vi "Low Pass Filter.vi"(0 "input signal":waveform(dbl)={"t0"=timestamp(0 s since 1904-01-01), "dt"=0.0, "Y"=[]}, 1 "Lower Cutoff Frequency (Hz)":dbl=1000.0 format="%#_15g", 3 "Upper Cutoff Frequency (Hz)":dbl=200.0 format="%#_15g", 5 "error in":errorcluster, 7 "reset":bool) -> (14 "filtered data":waveform(dbl), 19 "error out":errorcluster)   [LabVIEW 2014]
doc: "Filters a time signal using an infinite impulse response (IIR) or finite impulse response (FIR) filter. Use this step to remove or attenuate unwanted frequencies from a signal using various standard filter types and topologies.\n\nThis Express VI filters the input signal continuously. The Express VI resets the signal to its original value the first time the Express VI runs, if LabVIEW detects a discontinuity in the input signal, or if the <b>reset</b> input receives a TRUE value."
uses:
  <vilib>/measure/macond.llb/IIR Filter for 1 Chan.vi
  <vilib>/measure/NI_MAPro.lvlib
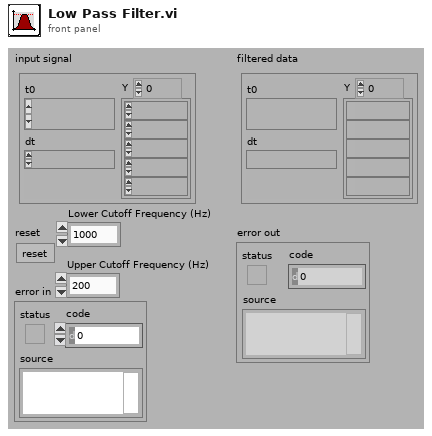
[diagram p1: front panel]
types:
  T1 = cluster{"Topology":enum16{"Off", "Butterworth", "Chebyshev", "Inverse Chebyshev", "Elliptic", "Bessel"}, "Type":enum16{"Lowpass", "Highpass", "Bandpass", "Bandstop"}, "Order":i32, "Lower Fc":dbl, "Upper Fc":dbl, "PB Ripple":dbl, "SB Attenuation":dbl}
  T2 = cluster{"Lower PB":dbl, "Upper PB":dbl, "Lower SB":dbl, "Upper SB":dbl, "PB Gain":dbl, "SB Gain":dbl, "Scale":bool}
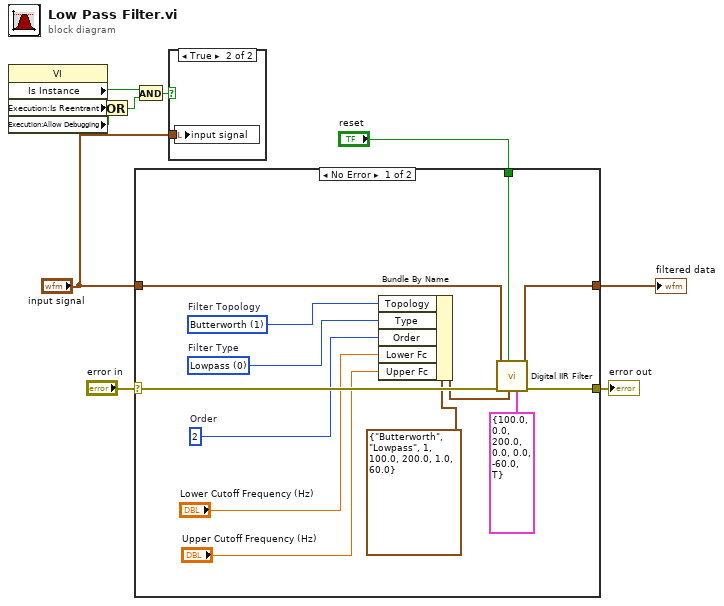
[diagram p0: block diagram]
diagram:
  n1 = property class="VI"() -> ("Is Instance"=w6:bool, "Execution:Is Reentrant"=w4:bool, "Execution:Allow Debugging"=w3:bool)  [unwired: 2 in, 2 out]
  n2 = Or(x=w4, y=w3) -> (x .or. y?=w5:bool)
  n3 = case shown="No Error" "error in" {
    selector: "error in" -> [w20 w24]
    tunnel: [w23 w24] -> w10
    tunnel: [w22 _] -> w8
    tunnel: "input signal" -> [w21 _]
    tunnel: "reset" -> [w19 _]
    frame No Error {
      w16 = u32 2  # Order
      w17 = u16 0 items=["Lowpass", "Highpass", "Bandpass", "Bandstop"]  # Filter Type
      w18 = u16 1 items=["Off", "Butterworth", "Chebyshev", "Inverse Chebyshev", "Elliptic", "Bessel"]  # Filter Topology
      n4 = Bundle By Name(cluster=T1 {"Topology"=enum."Butterworth", "Type"=enum."Lowpass", "Order"=1, "Lower Fc"=100.0, "Upper Fc"=200.0, "PB Ripple"=1.0, "SB Attenuation"=60.0} ("IIR filter specifications"), "Topology"=w18, "Type"=w17, "Order"=w16, "Lower Fc"="Lower Cutoff Frequency (Hz)", "Upper Fc"="Upper Cutoff Frequency (Hz)") -> (w12:T1)
      n5 = call-poly <vilib>:"Digital IIR Filter.vi"("optional IIR filter specifications"=T2 {"Lower PB"=100.0, "Upper PB"=0.0, "Lower SB"=200.0, "Upper SB"=0.0, "PB Gain"=0.0, "SB Gain"=-60.0, "Scale"=TRUE}, "IIR filter specifications"=w12, "reset filter"=w19, "error in (no error)"=w20, "signal in"=w21) -> ("error out"=w23:errorcluster, "signal out"=w22:waveform(dbl))  [unwired: 4 in, 1 out]
    }
    frame Error {
    }
  }
  "error out" <- w10
  "filtered data" <- w8
  n6 = And(x=w6, y=w5) -> (x .and. y?=w2:bool)
  n7 = case shown="True" w2 {
    tunnel: "input signal" -> [_ w25]
    frame False {
    }
    frame True {
      n8 = local write "input signal"(w25) -> ()
    }
  }
